vi "Trigger-hardware.vi"(8 "error in (no error)":errorcluster, 9 "Wakeup Reason":T1, 10 "Config. params. ref. in":refnum<data-value>, 11 "Acquis. params. ref. in":refnum<data-value>) -> (0 "error out":errorcluster, 1 "Tigger ok?":bool, 2 "Config. params. ref.":refnum<data-value>, 3 "Acquis. params. ref.":refnum<data-value>)   [LabVIEW 2013, in "CameraVision.lvlib" / "CV-Acquisition.lvclass"]
uses:
  CV-Acquisition.lvclass
  Configuration/CV-Configuration.lvclass
  <vilib>/Platform/TimedLoop/XDataNode/wakeup.ctl
  CV-Acquisition.lvclass/CV-Acquisition.ctl
  Configuration/CV-Configuration.lvclass/CV-Configuration.ctl
  Configuration/Read Framegrabber DLL file.vi
  Configuration/Read BoardHandle.vi
  Configuration/Read Camport array.vi
  <vilib>/DAQmx/read.llb/DAQmx Read (Digital Bool 1Line 1Point).vi
  Read Gate when.vi
  Read Gate source.vi
  Read Trigger mode.vi
  <vilib>/DAQmx/miscellaneous.llb/DAQmx Fill In Error Info.vi
  <vilib>/Platform/TimedLoop/XDataNode/XDNodeRunTimeDep.lvlib
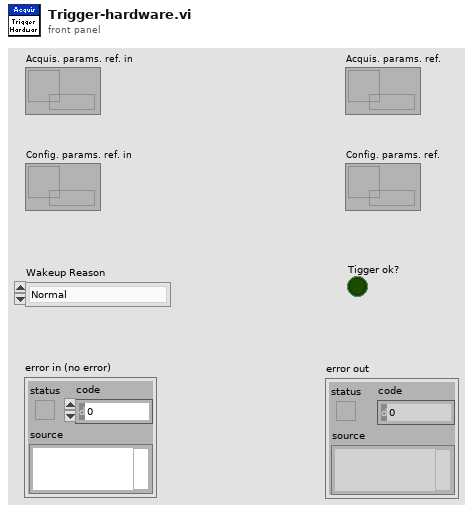
[diagram p1: front panel]
types:
  T1 = typedef "XDNodeRunTimeDep.lvlib/wakeup.ctl" = enum32{"Normal", "Aborted", "Asynchronous wakeup", "Timing source error", "Timed loop error", "Timeout"}
  T2 = typedef "Acquisition.lvclass/Trigger-modes.ctl" = enum16{"Camera timed (not sync.)", "Framegrabber timed (sync.)", "Software timed (sync.)", "External timing (sync.)", "Manual (sync.)", "Gated - camera (not sync.)", "Gated - grabber (sync.)", "Gated - software (sync.)", "Gated - external (sync.)"}
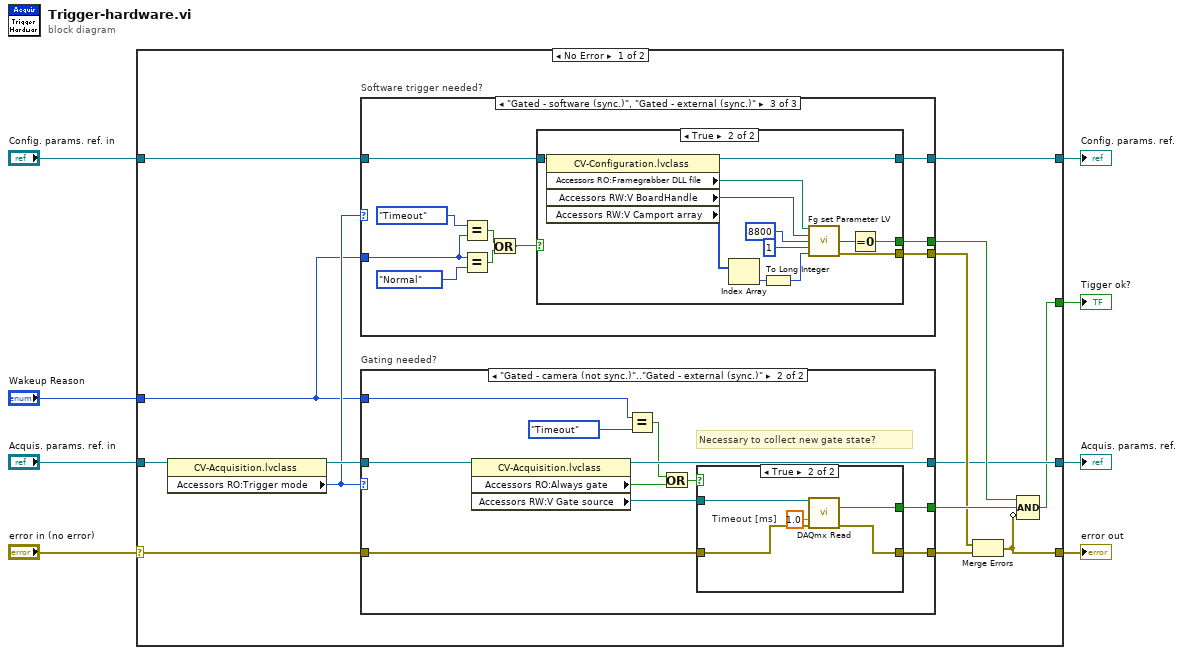
[diagram p0: block diagram]
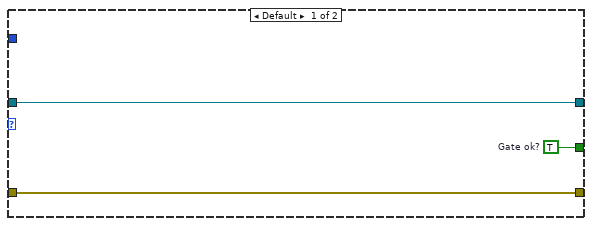
[diagram p2: hidden frame]
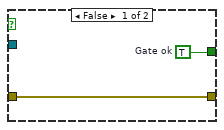
[diagram p3: hidden frame]
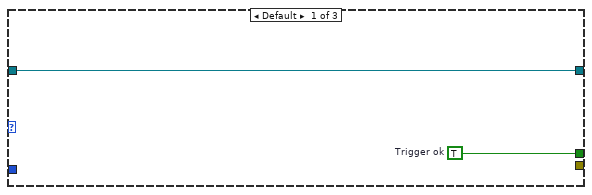
[diagram p4: hidden frame]
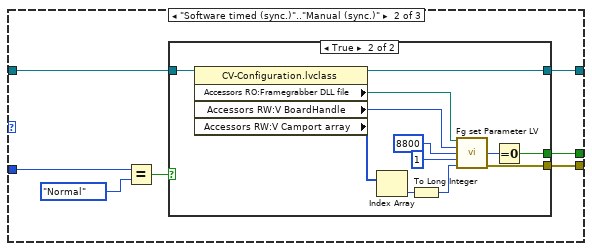
[diagram p5: hidden frame]
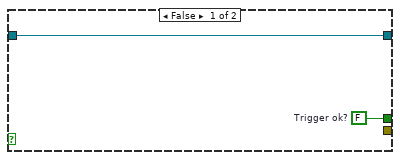
[diagram p6: hidden frame]
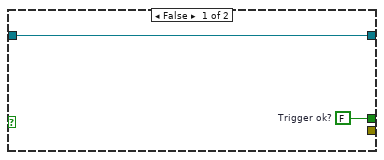
[diagram p7: hidden frame]
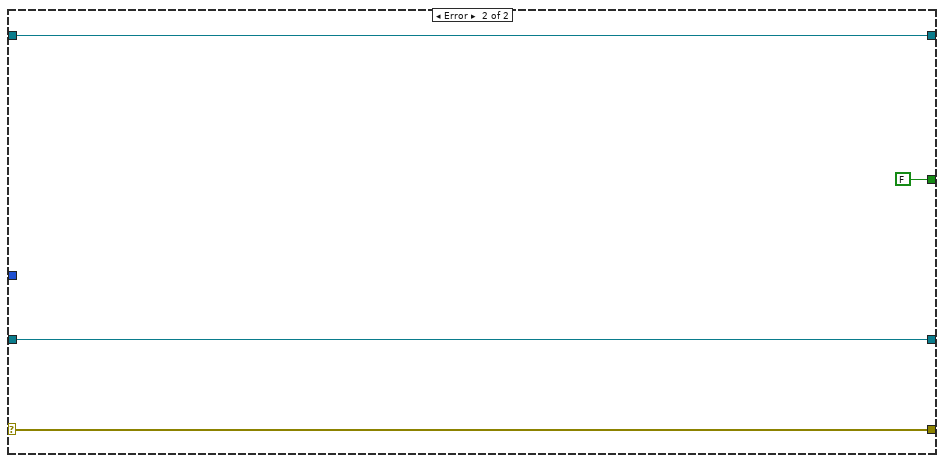
[diagram p8: hidden frame]
diagram:
  n1 = case shown="No Error" "error in (no error)" {
    selector: "error in (no error)" -> [w19 w94]
    tunnel: [w14 w94] -> w7
    tunnel: "Acquis. params. ref. in" -> [w22 w92]
    tunnel: [w13 w92] -> w3
    tunnel: [w12 w93] -> w4
    tunnel: "Config. params. ref. in" -> [w21 w93]
    tunnel: [w11 FALSE] -> w2
    tunnel: "Wakeup Reason" -> [w9 _]
    frame No Error {
      n2 = property class="CV-Acquisition.lvclass"(reference=w22) -> (reference out=w20:refnum<data-value>, "Accessors RO:Trigger mode"=w10:T2)  [unwired: 1 in, 1 out]
      n3 = case "Software trigger needed?" shown="\"Gated - software (sync.)\", \"Gated - external (sync.)\"" w10 {
        tunnel: w21 -> [w44 w52 w76]
        tunnel: [_ w51 w75] -> w15
        tunnel: [w45 w50 w74] -> w17
        tunnel: [w44 w49 w73] -> w12
        tunnel: w9 -> [_ w47 w71]
        frame Default {
          w45 = TRUE  # Trigger ok
        }
        frame "Software timed (sync.)".."Manual (sync.)" {
          n4 = Equal?(x=w47, y=wakeup."Normal") -> (x = y?=w46:bool)
          n5 = case shown="True" w46 {
            tunnel: w52 -> [w54 w66]
            tunnel: [_ w59] -> w51
            tunnel: [w53 w57] -> w50
            tunnel: [w54 w56] -> w49
            frame False {
              w53 = FALSE  # Trigger ok?
            }
            frame True {
              n6 = property class="CV-Configuration.lvclass"(reference=w66) -> (reference out=w56:refnum<data-value>, "Accessors RO:Framegrabber DLL file"=w60:path, "Accessors RW:V BoardHandle"=w55:u64, "Accessors RW:V Camport array"=w65:u32[])  [unwired: 1 in, 1 out]
              n7 = Index Array(array=w65) -> (element=w64:u32)  [unwired: 1 in]
              n8 = To Long Integer(number=w64) -> (32bit integer=w63:i32)
              n9 = call <userlib>:"Fg set Parameter LV.vi"("dll path in"=w60, "FgAddr"=w55, "Parameter"=8800, "Value"=u32 1, "CamPort"=w63) -> ("function return"=w58:i32, "error out"=w59:errorcluster)  [unwired: 8 in, 1 out]
              n10 = Equal To 0?(x=w58) -> (x = 0?=w57:bool)
            }
          }
        }
        frame "Gated - software (sync.)", "Gated - external (sync.)" {
          n11 = Equal?(x=wakeup."Timeout" ("y"), y=w71) -> (x = y?=w68:bool)
          n12 = Equal?(x=w71, y=wakeup."Normal") -> (x = y?=w69:bool)
          n13 = Or(x=w68, y=w69) -> (x .or. y?=w67:bool)
          n14 = case shown="True" w67 {
            tunnel: w76 -> [w78 w90]
            tunnel: [_ w83] -> w75
            tunnel: [w77 w81] -> w74
            tunnel: [w78 w80] -> w73
            frame False {
              w77 = FALSE  # Trigger ok?
            }
            frame True {
              n15 = property class="CV-Configuration.lvclass"(reference=w90) -> (reference out=w80:refnum<data-value>, "Accessors RO:Framegrabber DLL file"=w84:path, "Accessors RW:V BoardHandle"=w79:u64, "Accessors RW:V Camport array"=w89:u32[])  [unwired: 1 in, 1 out]
              n16 = Index Array(array=w89) -> (element=w88:u32)  [unwired: 1 in]
              n17 = To Long Integer(number=w88) -> (32bit integer=w87:i32)
              n18 = call <userlib>:"Fg set Parameter LV.vi"("dll path in"=w84, "FgAddr"=w79, "Parameter"=8800, "Value"=u32 1, "CamPort"=w87) -> ("function return"=w82:i32, "error out"=w83:errorcluster)  [unwired: 8 in, 1 out]
              n19 = Equal To 0?(x=w82) -> (x = 0?=w81:bool)
            }
          }
        }
      }
      n20 = case "Gating needed?" shown="\"Gated - camera (not sync.)\"..\"Gated - external (sync.)\"" w10 {
        tunnel: w20 -> [w24 w36]
        tunnel: w19 -> [w25 w35]
        tunnel: [w25 w34] -> w18
        tunnel: [w23 w33] -> w16
        tunnel: [w24 w32] -> w13
        tunnel: w9 -> [_ w30]
        frame Default {
          w23 = TRUE  # Gate ok?
        }
        frame "Gated - camera (not sync.)".."Gated - external (sync.)" {
          # "Necessary to collect new gate state?"
          n21 = property class="CV-Acquisition.lvclass"(reference=w36) -> (reference out=w32:refnum<data-value>, "Accessors RO:Always gate"=w27:bool, "Accessors RW:V Gate source"=w31:refnum<k21>)  [unwired: 1 in, 1 out]
          n22 = Equal?(x=w30, y=wakeup."Timeout") -> (x = y?=w28:bool)
          n23 = Or(x=w28, y=w27) -> (x .or. y?=w26:bool)
          n24 = case shown="True" w26 {
            tunnel: w35 -> [w37 w42]
            tunnel: [w37 w41] -> w34
            tunnel: [w38 w40] -> w33
            tunnel: w31 -> [_ w39]
            frame False {
              w38 = TRUE  # Gate ok
            }
            frame True {
              w43 = 1.0  # Timeout [ms]
              n25 = call-poly <vilib>:"DAQmx Read.vi"("task/channels in"=w39, "timeout"=w43, "error in"=w42) -> ("data"=w40:bool, "error out"=w41:errorcluster)  [unwired: 10 in, 1 out]
            }
          }
        }
      }
      n26 = Merge Errors(w15, w18) -> (w14:errorcluster)
      n27 = Compound Arithmetic op=AND(w17, w16, invert w14) -> (w11:bool)
    }
    frame Error {
    }
  }
  "error out" <- w7
  "Acquis. params. ref." <- w3
  "Config. params. ref." <- w4
  "Tigger ok?" <- w2
